vi "DSF.Engine.Interface.Transceiver.Read.Error.vi"(8 "error in (no error)":errorcluster, 9 "timeout in ms (0)":i32 format="%d ms", 11 "Transceiver Interface in":refnum<class "DSF.Engine.Interface.Transceiver.lvclass">) -> (0 "error out":errorcluster, 1 "empty?":bool, 2 "error":errorcluster, 3 "Transceiver Interface out":refnum<class "DSF.Engine.Interface.Transceiver.lvclass">)   [LabVIEW 2017, in "Data Sharing Framework Engine.lvlib" / "DSF.Engine.Interface.Transceiver.lvclass"]
uses:
  DSF.Engine.Interface.Transceiver.lvclass
  C:/github/data-sharing-framework/old/dsf core/Source/Engine/Classes/Interface/DSF.Engine.Interface.lvclass
  DSF.Engine.Interface.lvclass/DSF.Engine.Interface.ctl
  DSF.Engine.Interface.Get Debug Flags.vi
  DSF.Engine.Interface.Get Error Queue.vi
  DSF.Engine.Interface.Error Queue.Read.vi
  DSF.Engine.Interface.lvclass
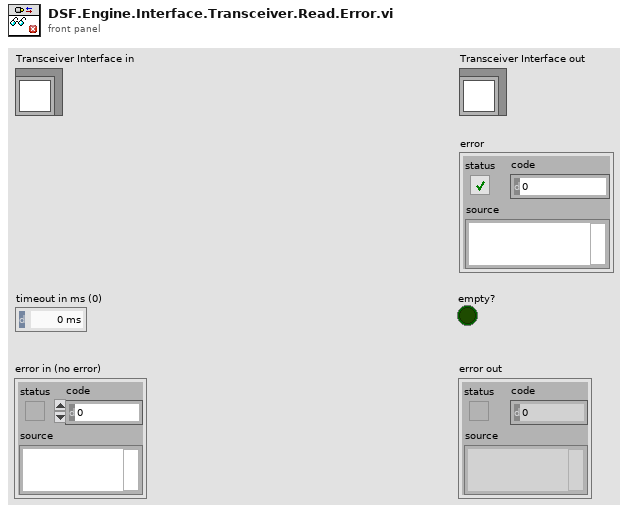
[diagram p1: front panel]
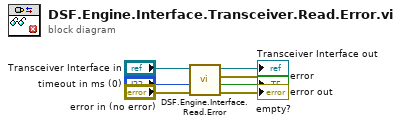
[diagram p0: block diagram]
diagram:
  n1 = call "DSF.Engine.Interface.Read.Error.vi"("error in (no error)"="error in (no error)", "timeout in ms (0)"="timeout in ms (0)", "Interface in"="Transceiver Interface in") -> ("error out"=→"error out":errorcluster, "timed out?"=→"empty?":bool, "error"=→"error":errorcluster, "Interface out"=→"Transceiver Interface out":refnum<class "DSF.Engine.Interface.Transceiver.lvclass">)  [unwired: 5 in]
